vi "Modify Data format to R2_filled.vi"(6 "Current set number in one current mode":i32=48, 7 "Scan number":i32=10, 8 "modified error":errorcluster, 9 "modified Data path":path, 10 "original error":errorcluster, 11 "original Data path":path) -> ()   [LabVIEW 2023]
uses:
  <vilib>/Utility/error.llb/DialogType.ctl
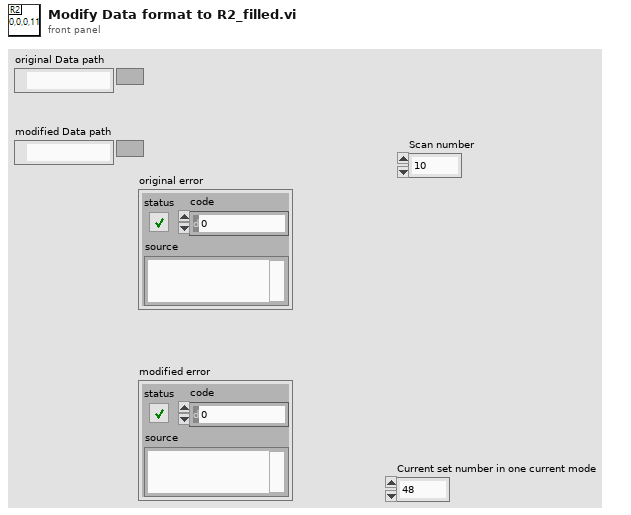
[diagram p1: front panel]
types:
  T1 = enum16{"open", "replace", "create", "open or create", "replace or create", "replace or create with confirmation"}
  T2 = typedef "DialogType.ctl" = u16
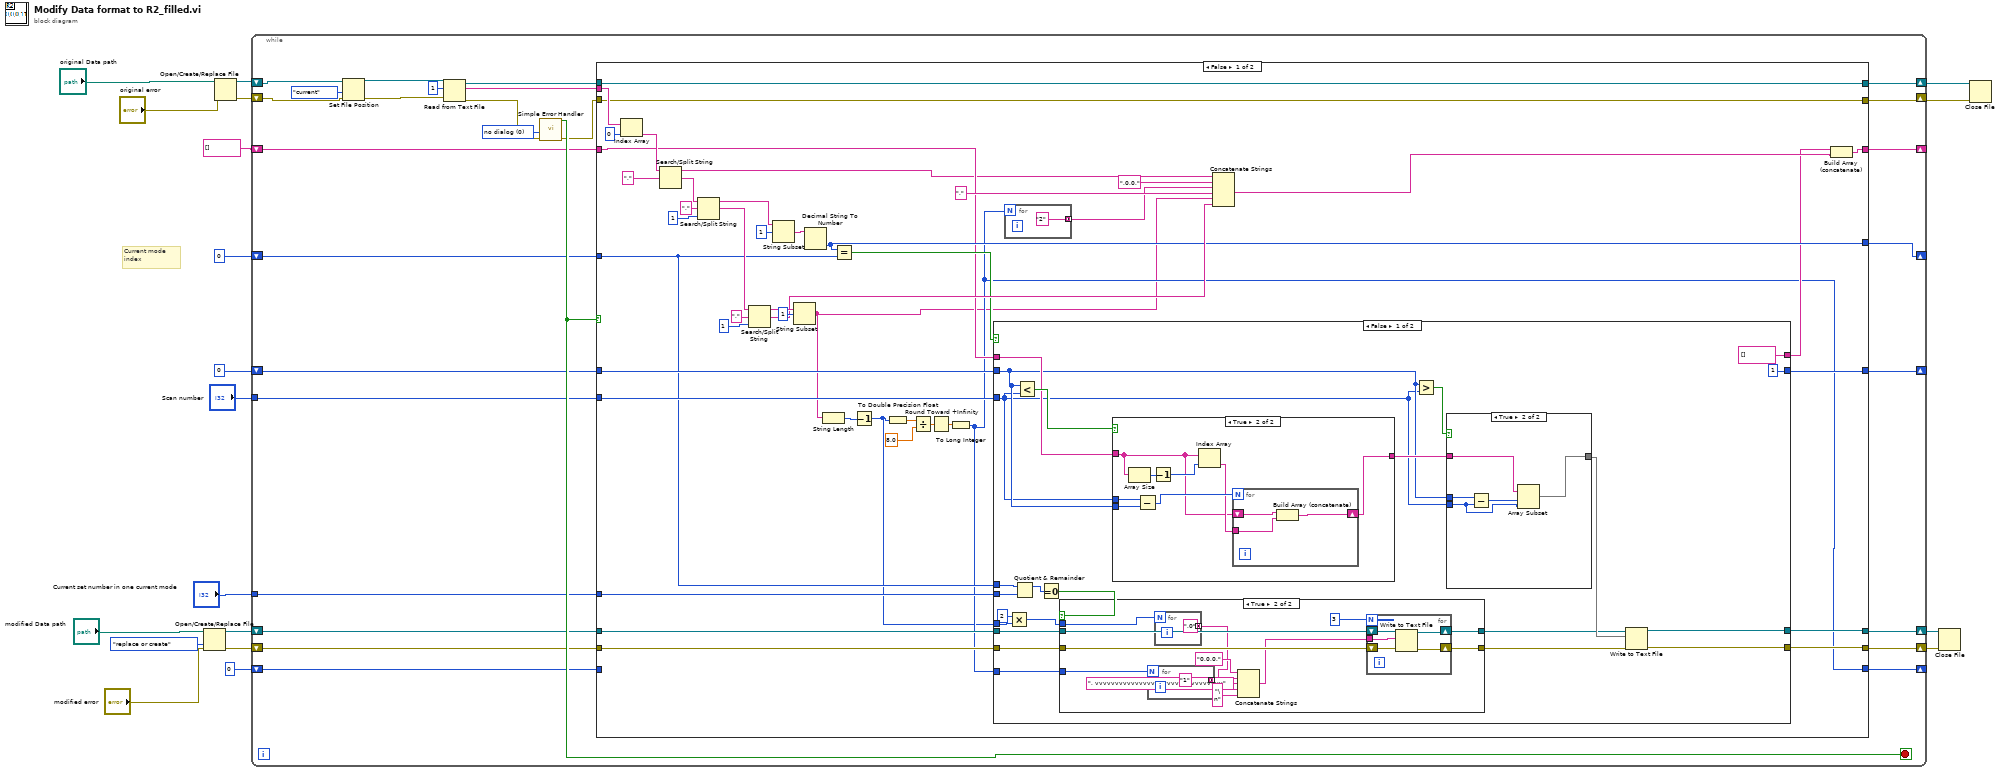
[diagram p0: block diagram]
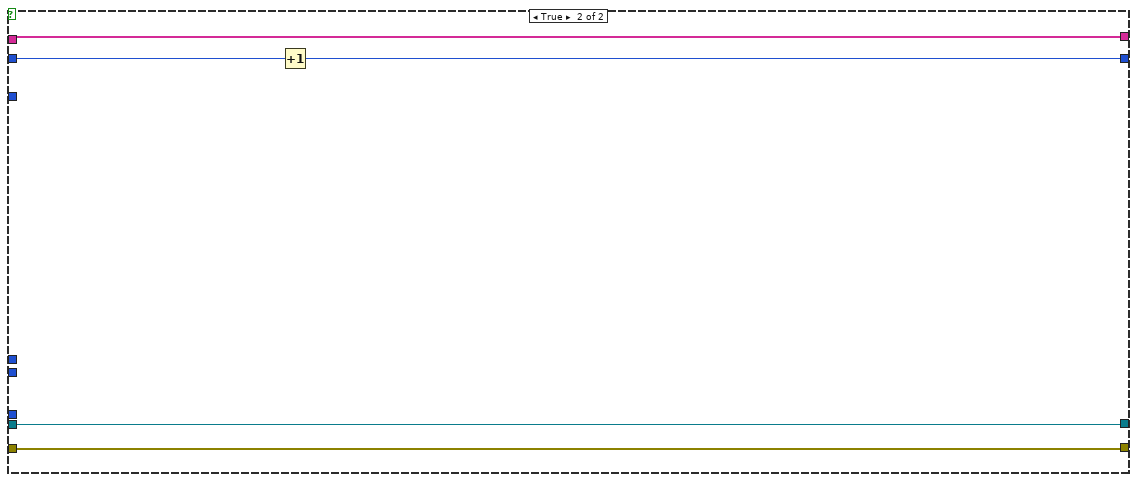
[diagram p5: hidden frame]
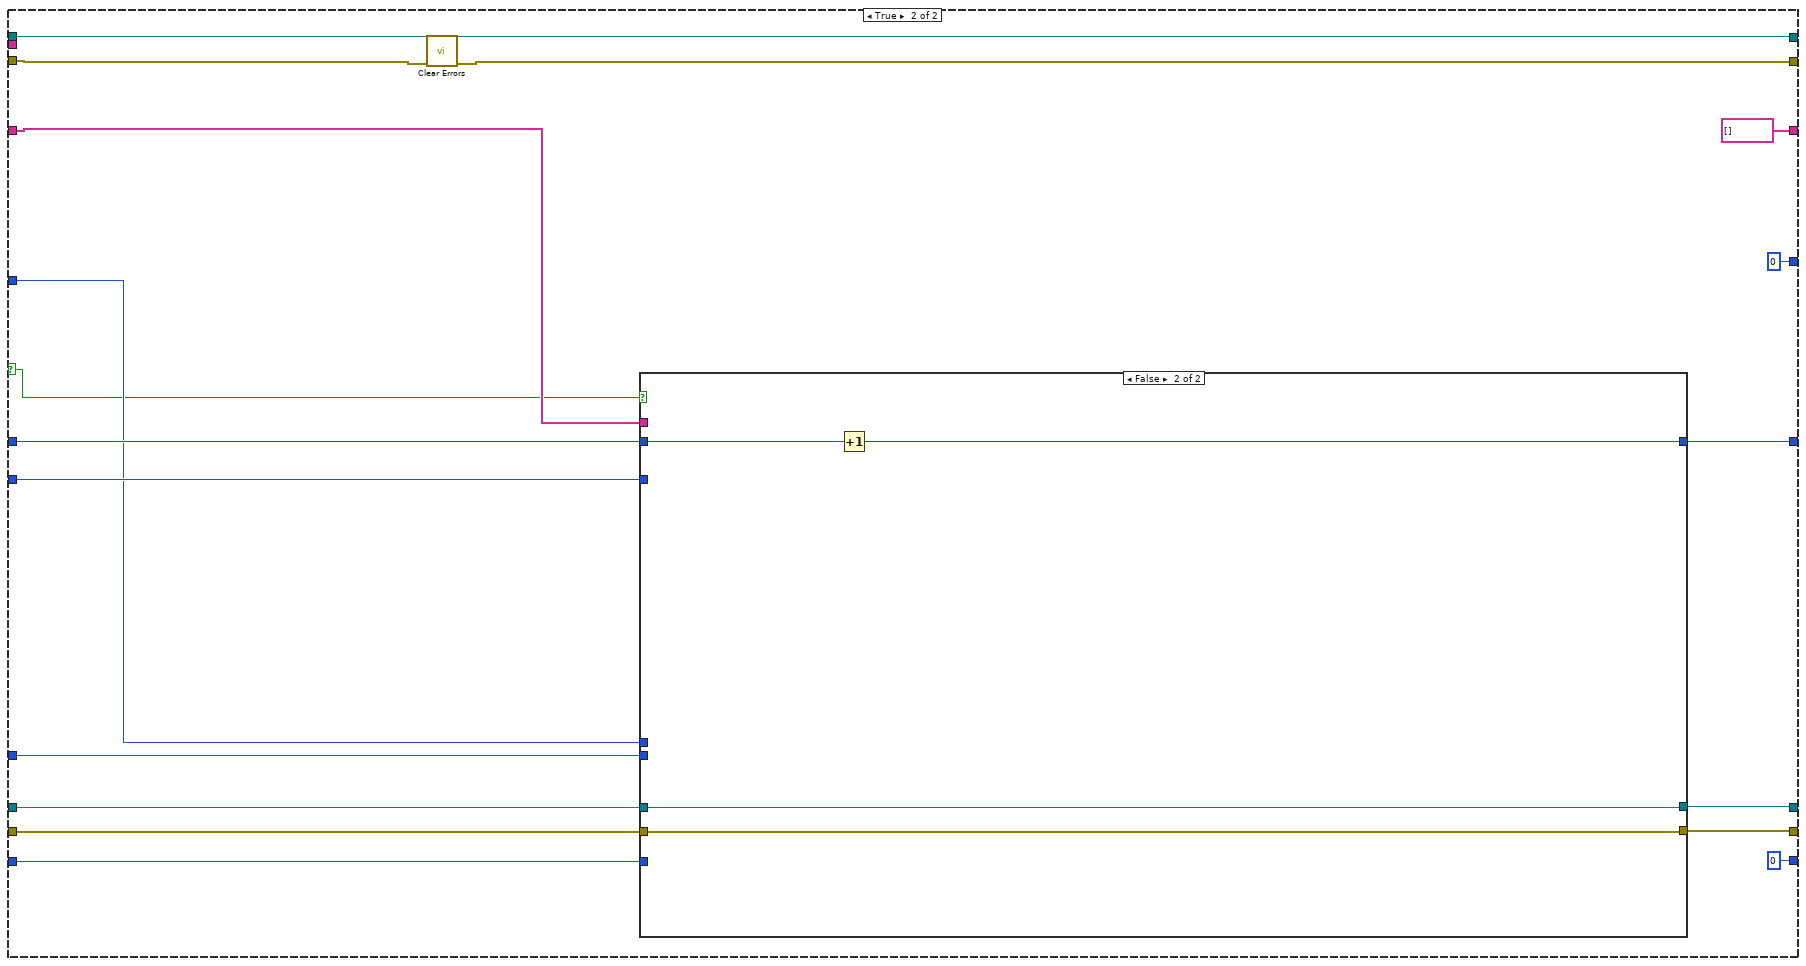
[diagram p6: hidden frame]
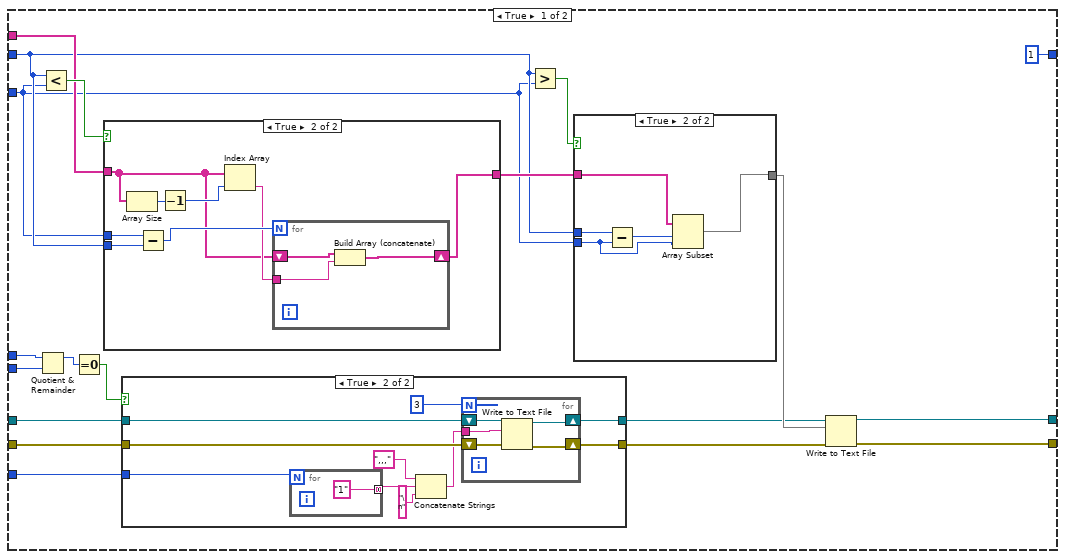
[diagram p7: hidden frame]
diagram:
  # "Current mode\nindex"
  n1 = Open/Create/Replace File(file path (use dialog)="modified Data path", error in="modified error", operation (0:open)=T1."replace or create") -> (refnum out=w16:refnum<file>, error out=w15:errorcluster)  [unwired: 3 in, 1 out]
  n2 = Open/Create/Replace File(file path (use dialog)="original Data path", error in="original error") -> (refnum out=w17:refnum<file>, error out=w18:errorcluster)  [unwired: 4 in, 1 out]
  n3 = while {
    shift-right: [w39] -> w9
    shift-left: w18 -> [w46]
    shift-right: [w38] -> w19
    shift-left: w17 -> [w37]
    shift-right: [w32] -> w11
    shift-left: w16 -> [w34]
    shift-right: [w31] -> w10
    shift-left: w15 -> [w33]
    shift-right: [w20] -> _
    shift-left: string[] [] ("element") -> [w29]
    shift-right: [w25] -> _
    shift-left: 0 ("number") -> [w28]
    shift-right: [w26] -> _
    shift-left: 0 ("number") -> [w27]
    tunnel: "Scan number" -> [w24]
    tunnel: "Current set number in one current mode" -> [w23]
    shift-right: [w22] -> _
    shift-left: 0 ("32bit integer") -> [w21]
    stop <- w43 stop-if-true
    w44 = T2 0 items=["no dialog", "OK message", "continue or stop message", "OK message + warnings", "continue/stop + warnings"] ("type of dialog (OK msg:1)")
    n4 = Set File Position(refnum=w37, from (0:start)=enum16{"start", "end", "current"}."current", error in=w46) -> (refnum out=w36:refnum<file>, error out=w35:errorcluster)  [unwired: 1 in]
    n5 = Read from Text File(file (use dialog)=w36, count=1, error in=w35) -> (refnum out=w41:refnum<file>, text=w42:string[], error out=w40:errorcluster)  [unwired: 1 in, 1 out]
    n6 = call <vilib>:"Simple Error Handler.vi"("type of dialog (OK msg:1)"=w44, "error in (no error)"=w40) -> ("error?"=w43:bool, "error out"=w30:errorcluster)  [unwired: 3 in, 3 out]
    n7 = case shown="False" w43 {
      selector: w43 -> [_ w166]
      tunnel: w42 -> [w87 _]
      tunnel: w41 -> [w85 w179]
      tunnel: w30 -> [w84 w168]
      tunnel: [w85 w179] -> w38
      tunnel: [w84 w167] -> w39
      tunnel: w34 -> [w65 w174]
      tunnel: w33 -> [w64 w173]
      tunnel: [w63 w172] -> w32
      tunnel: [w62 w171] -> w31
      tunnel: w29 -> [w67 w175]
      tunnel: w28 -> [w61 w170]
      tunnel: w27 -> [w72 w178]
      tunnel: [w71 w177] -> w26
      tunnel: [w70 0] -> w25
      tunnel: w24 -> [w68 w176]
      tunnel: w23 -> [w60 w169]
      tunnel: [w52 0] -> w22
      tunnel: w21 -> [_ w163]
      tunnel: [w51 string[] [] ("element")] -> w20
      frame False {
        n8 = Index Array(array=w87, index=0) -> (element=w83:string)
        n9 = Search/Split String(string=w83, search string/char (-)=",") -> (substring before match=w55:string, match + rest of string=w92:string)  [unwired: 1 in, 1 out]
        n10 = Search/Split String(string=w92, search string/char (-)=",", offset (0)=1) -> (substring before match=w75:string, match + rest of string=w80:string)  [unwired: 1 out]
        n11 = Search/Split String(string=w80, search string/char (-)=",", offset (0)=1) -> (substring before match=w79:string, match + rest of string=w77:string)  [unwired: 1 out]
        n12 = String Subset(string=w75, offset (0)=1) -> (substring=w74:string)  [unwired: 1 in]
        n13 = String Subset(string=w79, offset (0)=1) -> (substring=w50:string)  [unwired: 1 in]
        n14 = Decimal String To Number(string=w74) -> (number=w70:i32)  [unwired: 2 in, 1 out]
        n15 = String Length(string=w50) -> (length=w49:i32)
        n16 = Equal?(x=w70, y=w61) -> (x = y?=w73:bool)
        n17 = Decrement(x=w49) -> (x-1=w48:i32)
        n18 = To Double Precision Float(number=w48) -> (double precision float=w58:dbl)
        n19 = Divide(x=w58, y=8.0) -> (x/y=w59:dbl)
        n20 = Round Toward +Infinity(x=w59) -> (ceil(x): smallest int >= x=w56:dbl)
        n21 = To Long Integer(number=w56) -> (32bit integer=w52:i32)
        n22 = case shown="False" w73 {
          tunnel: [1 w160] -> w71
          tunnel: w72 -> [w110 w161]
          tunnel: w68 -> [w109 _]
          tunnel: w67 -> [w113 w159]
          tunnel: [string[] [] ("element") w159] -> w66
          tunnel: w65 -> [w101 w158]
          tunnel: w64 -> [w100 w157]
          tunnel: [w107 w158] -> w63
          tunnel: [w106 w157] -> w62
          tunnel: w61 -> [w105 _]
          tunnel: w60 -> [w104 _]
          tunnel: w52 -> [w97 _]
          tunnel: w48 -> [w96 _]
          frame False {
            n23 = Multiply(x=2, y=w96) -> (x*y=w94:i32)
            n24 = Quotient & Remainder(x=w105, y=w104) -> (x-y*floor(x/y)=w103:i32)  [unwired: 1 out]
            n25 = Less?(x=w110, y=w109) -> (x < y?=w114:bool)
            n26 = Equal To 0?(x=w103) -> (x = 0?=w102:bool)
            n27 = case shown="True" w102 {
              tunnel: w101 -> [w118 w128]
              tunnel: w100 -> [w117 w127]
              tunnel: [w118 w125] -> w99
              tunnel: [w117 w124] -> w98
              tunnel: w97 -> [_ w123]
              tunnel: w94 -> [_ w122]
              frame False {
              }
              frame True {
                n28 = for {
                  N: w123 -> [_]
                  tunnel: ["1" ("search string/char (-)")] -> w130 mode=concatenating
                }
                n29 = for {
                  N: w122 -> [_]
                  tunnel: [",0" ("search string/char (-)")] -> w121 mode=concatenating
                }
                n30 = Concatenate Strings("0,0,0," ("string"), w130, ", vvvvvvvvvvvvvvvvvvvvvvvvvvvvvvvv" ("string"), w121, "\n" ("string")) -> (w126:string)
                n31 = for {
                  N: 3 -> [_]
                  shift-right: [w135] -> w125
                  shift-left: w128 -> [w138]
                  tunnel: w126 -> [w136]
                  shift-right: [w134] -> w124
                  shift-left: w127 -> [w137]
                  n32 = Write to Text File(file (use dialog)=w138, text=w136, error in=w137) -> (refnum out=w135:refnum<file>, error out=w134:errorcluster)  [unwired: 1 in, 1 out]
                }
              }
            }
            n33 = case shown="True" w114 {
              tunnel: w113 -> [w145 w147]
              tunnel: w109 -> [_ w151]
              tunnel: w110 -> [_ w150]
              tunnel: [w145 w146] -> w111
              frame False {
              }
              frame True {
                n34 = Array Size(array=w147) -> (size(s)=w153:i32)
                n35 = Subtract(x=w151, y=w150) -> (x-y=w149:i32)
                n36 = Decrement(x=w153) -> (x-1=w152:i32)
                n37 = Index Array(array=w147, index=w152) -> (element=w148:string)
                n38 = for {
                  N: w149 -> [_]
                  tunnel: w148 -> [w154]
                  shift-right: [w155] -> w146
                  shift-left: w147 -> [w156]
                  n39 = Build Array (concatenate)(w156, w154) -> (w155:string[])
                }
              }
            }
            n40 = Greater?(x=w110, y=w109) -> (0:w112:bool)
            n41 = case shown="True" w112 {
              tunnel: w111 -> [w139 w143]
              tunnel: w110 -> [_ w144]
              tunnel: w109 -> [_ w141]
              tunnel: [w139 w140] -> w108
              frame False {
              }
              frame True {
                n42 = Subtract(x=w144, y=w141) -> (x-y=w142:i32)
                n43 = Array Subset(array=w143, index=w142, length=w141) -> (w140:string[])
              }
            }
            n44 = Write to Text File(file (use dialog)=w99, text=w108, error in=w98) -> (refnum out=w107:refnum<file>, error out=w106:errorcluster)  [unwired: 1 in, 1 out]
          }
          frame True {
            n45 = Increment(x=w161) -> (x+1=w160:i32)
          }
        }
        n46 = for {
          N: w52 -> [_]
          tunnel: ["2" ("search string/char (-)")] -> w53 mode=concatenating
        }
        n47 = Concatenate Strings(w55, ",0,0," ("string"), w53, "," ("string"), w50, w77) -> (w69:string)
        n48 = Build Array (concatenate)(w66, w69) -> (w51:string[])
      }
      frame True {
        n49 = call <vilib>:"Clear Errors.vi"("error in (no error)"=w168) -> ("error out"=w167:errorcluster)  [unwired: 5 in, 1 out]
        n50 = case shown="False" w166 {
          tunnel: [1 w237] -> w177
          tunnel: w178 -> [w193 w238]
          tunnel: w176 -> [w192 _]
          tunnel: w175 -> [w196 _]
          tunnel: w174 -> [w184 w236]
          tunnel: w173 -> [w183 w235]
          tunnel: [w190 w236] -> w172
          tunnel: [w189 w235] -> w171
          tunnel: w170 -> [w188 _]
          tunnel: w169 -> [w187 _]
          tunnel: w163 -> [w180 _]
          frame True {
            n51 = Quotient & Remainder(x=w188, y=w187) -> (x-y*floor(x/y)=w186:i32)  [unwired: 1 out]
            n52 = Less?(x=w193, y=w192) -> (x < y?=w197:bool)
            n53 = Equal To 0?(x=w186) -> (x = 0?=w185:bool)
            n54 = case shown="True" w197 {
              tunnel: w196 -> [w223 w225]
              tunnel: w192 -> [_ w229]
              tunnel: w193 -> [_ w228]
              tunnel: [w223 w224] -> w194
              frame False {
              }
              frame True {
                n55 = Array Size(array=w225) -> (size(s)=w231:i32)
                n56 = Subtract(x=w229, y=w228) -> (x-y=w227:i32)
                n57 = Decrement(x=w231) -> (x-1=w230:i32)
                n58 = Index Array(array=w225, index=w230) -> (element=w226:string)
                n59 = for {
                  N: w227 -> [_]
                  tunnel: w226 -> [w232]
                  shift-right: [w233] -> w224
                  shift-left: w225 -> [w234]
                  n60 = Build Array (concatenate)(w234, w232) -> (w233:string[])
                }
              }
            }
            n61 = case shown="True" w185 {
              tunnel: w184 -> [w200 w206]
              tunnel: w183 -> [w199 w205]
              tunnel: [w200 w203] -> w182
              tunnel: [w199 w202] -> w181
              tunnel: w180 -> [_ w201]
              frame False {
              }
              frame True {
                n62 = for {
                  N: w201 -> [_]
                  tunnel: ["1" ("search string/char (-)")] -> w209 mode=concatenating
                }
                n63 = Concatenate Strings(",,," ("string"), w209, "\n" ("string")) -> (w204:string)
                n64 = for {
                  N: 3 -> [_]
                  shift-right: [w213] -> w203
                  shift-left: w206 -> [w216]
                  tunnel: w204 -> [w214]
                  shift-right: [w212] -> w202
                  shift-left: w205 -> [w215]
                  n65 = Write to Text File(file (use dialog)=w216, text=w214, error in=w215) -> (refnum out=w213:refnum<file>, error out=w212:errorcluster)  [unwired: 1 in, 1 out]
                }
              }
            }
            n66 = Greater?(x=w193, y=w192) -> (0:w195:bool)
            n67 = case shown="True" w195 {
              tunnel: w194 -> [w217 w221]
              tunnel: w193 -> [_ w222]
              tunnel: w192 -> [_ w219]
              tunnel: [w217 w218] -> w191
              frame False {
              }
              frame True {
                n68 = Subtract(x=w222, y=w219) -> (x-y=w220:i32)
                n69 = Array Subset(array=w221, index=w220, length=w219) -> (w218:string[])
              }
            }
            n70 = Write to Text File(file (use dialog)=w182, text=w191, error in=w181) -> (refnum out=w190:refnum<file>, error out=w189:errorcluster)  [unwired: 1 in, 1 out]
          }
          frame False {
            n71 = Increment(x=w238) -> (x+1=w237:i32)
          }
        }
      }
    }
  }
  n72 = Close File(refnum=w11, error in=w10) -> ()  [unwired: 2 out]
  n73 = Close File(refnum=w19, error in=w9) -> ()  [unwired: 2 out]
